vi "User Config Get Path.vi"(8 "error in (no error)":errorcluster, 9 "filename":string="gscript_config.ini", 10 "Folder":string="gScript") -> (0 "error out":errorcluster, 3 "INI Path":path)   [LabVIEW 2024]
uses:
  <vilib>/Utility/sysdir.llb/System Directory Type.ctl
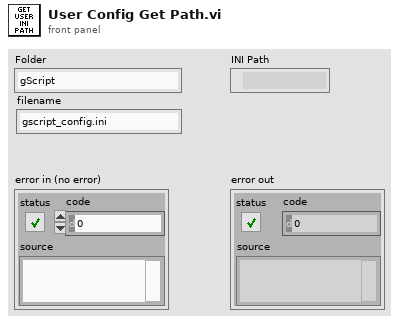
[diagram p1: front panel]
types:
  T1 = typedef "System Directory Type.ctl" = i32
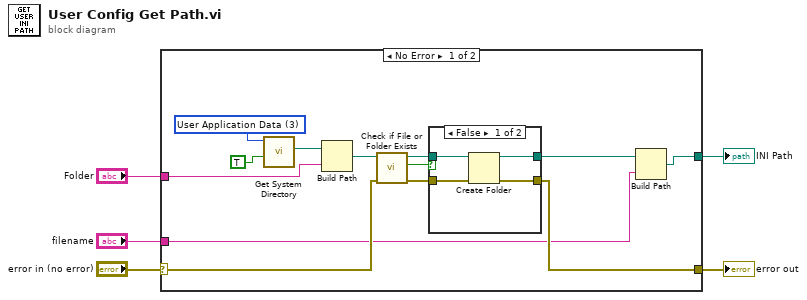
[diagram p0: block diagram]
diagram:
  n1 = case shown="No Error" "error in (no error)" {
    selector: "error in (no error)" -> [w11 w25]
    tunnel: [w10 w25] -> w2
    tunnel: [w8 _] -> w1
    tunnel: "Folder" -> [w7 _]
    tunnel: "filename" -> [w6 _]
    frame No Error {
      w17 = T1 3 items=["User Home"=0, "User Desktop"=1, "User Documents"=2, "User Application Data"=3, "User Preferences"=4, "User Temporary"=5, "Public Documents"=6, "Public Application Data"=7, "Public Preferences"=8, "Public Cache"=13, "System Core Libraries"=9, "System Installed Libraries"=10, "Application Files"=11, "Boot Volume Root"=12] ("system directory type")
      n2 = call <vilib>:"Get System Directory.vi"("create directory if not found? (F)"=TRUE, "system directory type"=w17) -> ("system directory"=w16:path)  [unwired: 9 in]
      n3 = Build Path(base path=w16, name or relative path=w7) -> (appended path=w15:path)
      n4 = call <vilib>:"Check if File or Folder Exists.vi"("error in (no error)"=w11, "path"=w15) -> ("error out"=w13:errorcluster, "file or folder exists?"=w14:bool, "dup path"=w12:path)  [unwired: 7 in]
      n5 = case shown="False" w14 {
        tunnel: w13 -> [w22 w23]
        tunnel: w12 -> [w21 w24]
        tunnel: [w20 w23] -> w10
        tunnel: [w19 w24] -> w9
        frame False {
          n6 = Create Folder(path (use dialog)=w21, error in=w22) -> (created path=w19:path, error out=w20:errorcluster)  [unwired: 1 in, 1 out]
        }
        frame True {
        }
      }
      n7 = Build Path(base path=w9, name or relative path=w6) -> (appended path=w8:path)
    }
    frame Error {
    }
  }
  "error out" <- w2
  "INI Path" <- w1
